vi "Instr_InitObject.vi"(8 "error in (no error)":errorcluster, 9 "Instrument Configuration":variant, 10 "Instrument address":refnum<visa-resource-name>, 11 "HP4263B in":refnum<class "HP4263B.lvclass">) -> (0 "error out":errorcluster, 3 "HP4263B out":refnum<class "HP4263B.lvclass">)   [LabVIEW 2013, in "HP4263B.lvclass"]
uses:
  HP4263B.lvclass
  LCRControl.lvclass
  InstrumentSetup.vi
  HP4263B_CommandsGlobal.vi
  InstrControl.lvclass
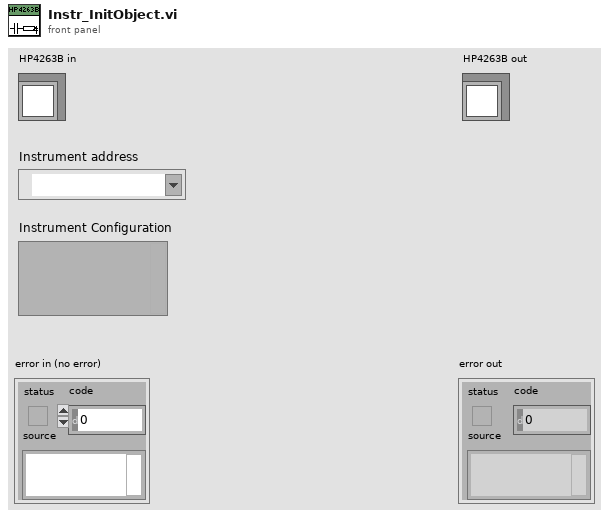
[diagram p1: front panel]
types:
  T1 = cluster{"RC Configuration":u16, "AC amplitude [V]":dbl, "AC frequency [Hz]":i32, "Cable Length":u16, "Averaging":u16, "Averaging Count":i32, "HP4263B":refnum<class "HP4263B.lvclass">}
  T2 = cluster{"Instrument name":string, "Instrument type":u16, "Command \"Initialise LCR\"":string, "Command \"OC Trim\"":string, "Command \"LCR Readout\"":string}
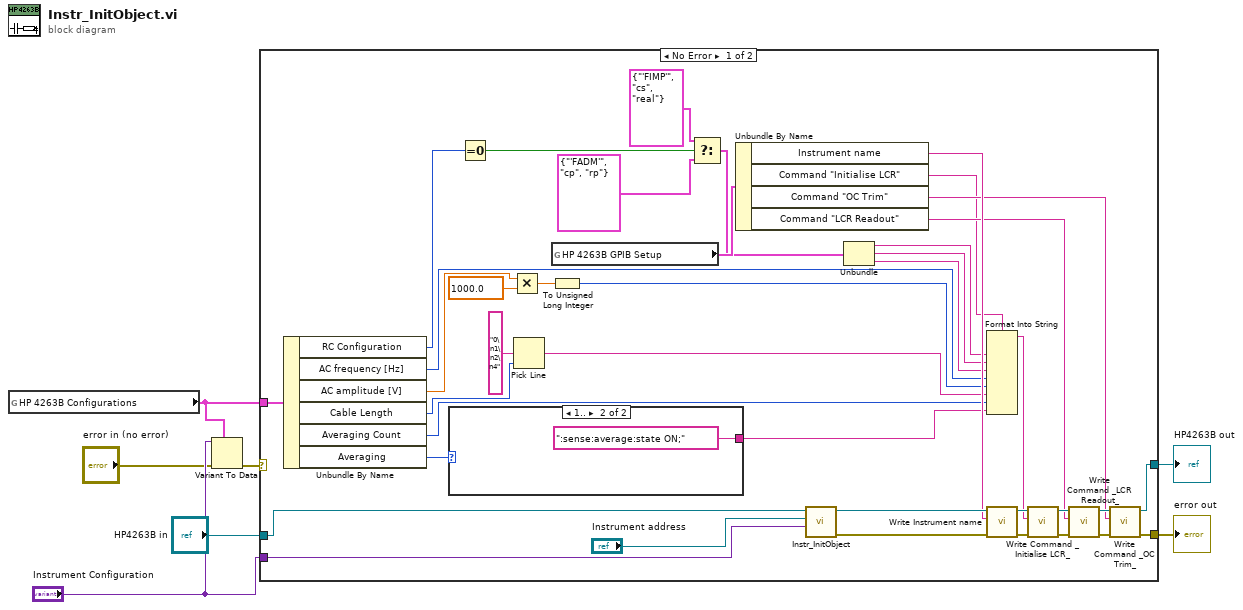
[diagram p0: block diagram]
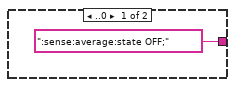
[diagram p2: hidden frame]
diagram:
  n1 = global read "InstrumentSetup.vi" "HP 4263B Configurations"() -> (w1:T1)
  n2 = Variant To Data(error in="error in (no error)", type=w1, Variant="Instrument Configuration") -> (error out=w2:errorcluster)  [unwired: 1 out]
  n3 = case shown="No Error" w2 {
    selector: w2 -> [_ w49]
    tunnel: "HP4263B in" -> [w44 w50]
    tunnel: [w33 w50] -> w6
    tunnel: [w32 w49] -> w5
    tunnel: "Instrument Configuration" -> [w46 _]
    tunnel: w1 -> [w29 _]
    frame No Error {
      n4 = Unbundle By Name(w29) -> ("RC Configuration"=w22:u16, "AC frequency [Hz]"=w14:i32, "AC amplitude [V]"=w26:dbl, "Cable Length"=w23:u16, "Averaging Count"=w10:i32, "Averaging"=w11:u16)
      n5 = case shown="1.." w11 {
        tunnel: [":sense:average:state OFF;" ":sense:average:state ON;"] -> w9
        frame ..0 {
        }
        frame 1.. {
        }
      }
      n6 = Equal To 0?(x=w22) -> (x = 0?=w21:bool)
      n7 = Multiply(x=w26, y=1000.0) -> (x*y=w28:dbl)
      n8 = Pick Line(multi-line string="0\n1\n2\n4", line index=w23) -> (output string=w12:string)  [unwired: 1 in]
      n9 = global read "HP4263B_CommandsGlobal.vi" "HP 4263B GPIB Setup"() -> (w43:T2)
      n10 = To Unsigned Long Integer(number=w28) -> (unsigned 32bit integer=w13:u32)
      n11 = Select(t=cluster{string, string, string} {"'FIMP'", "cs", "real"}, s=w21, f=cluster{string, string, string} {"'FADM'", "cp", "rp"}) -> (s? t:f=w18:cluster{string, string, string})
      n12 = Unbundle By Name(w43) -> ("Instrument name"=w40:string, "Command \"Initialise LCR\""=w25:string, "Command \"OC Trim\""=w31:string, "Command \"LCR Readout\""=w30:string)
      n13 = call-parent "Instr_InitObject.vi"("Instrument Configuration"=w46, "Instrument address"="Instrument address", "LCRControl in"=w44) -> ("error out"=w41:errorcluster, "LCRControl out"=w42:refnum<class "HP4263B.lvclass">)  [unwired: 7 in]
      n14 = Unbundle(w18) -> (w17:string, w16:string, w15:string)
      n15 = Format Into String(format string=w25, w17, w16, w15, w14, w13, w12, w10, w9) -> (resulting string=w8:string)  [unwired: 2 in, 1 out]
      n16 = call-dynamic "Write Instrument name.vi"("error in (no error)"=w41, "Instrument name"=w40, "InstControl in"=w42) -> ("error out"=w36:errorcluster, "InstControl out"=w37:refnum<class "HP4263B.lvclass">)  [unwired: 7 in]
      n17 = call-dynamic "Write Command _Initialise LCR_.vi"("error in (no error)"=w36, "Command \"Initialise LCR\""=w8, "LCRControl in"=w37) -> ("error out"=w38:errorcluster, "LCRControl out"=w35:refnum<class "HP4263B.lvclass">)  [unwired: 7 in]
      n18 = call-dynamic "Write Command _LCR Readout_.vi"("error in (no error)"=w38, "Command \"LCR Readout\""=w30, "LCRControl in"=w35) -> ("error out"=w39:errorcluster, "LCRControl out"=w34:refnum<class "HP4263B.lvclass">)  [unwired: 7 in]
      n19 = call-dynamic "Write Command _OC Trim_.vi"("error in (no error)"=w39, "Command \"OC Trim\""=w31, "LCRControl in"=w34) -> ("error out"=w32:errorcluster, "LCRControl out"=w33:refnum<class "HP4263B.lvclass">)  [unwired: 7 in]
    }
    frame Error {
    }
  }
  "error out" <- w5
  "HP4263B out" <- w6
